vi "DEMO.vi"() -> ()   [LabVIEW 2011]
panel:
  out "输出信息":string
  in  "输入信息":string
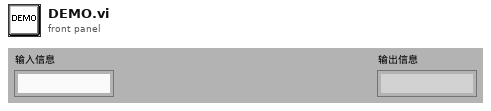
[diagram p1: front panel]
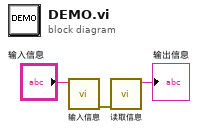
[diagram p0: block diagram]
diagram:
  n1 = call "输入信息.vi"("输入信息"="输入信息") -> ("error out"=w2:errorcluster)  [unwired: 10 in]
  n2 = call "读取信息.vi"("error in (no error)"=w2) -> ("输出信息"=→"输出信息":string)  [unwired: 9 in, 1 out]
